vi "TEMP MOVE BIAS.vi"(0 "ScanQ in":refnum<queue>, 2 "Translation":cluster{"x":dbl, "y":dbl}, 5 "x":dbl, 7 "Boolean":bool, 9 "y":dbl, 11 "error in (no error)":errorcluster) -> (4 "ScanQ out":refnum<queue>, 6 "X (m)":sgl, 10 "Y (m)":sgl, 15 "error out":errorcluster)   [LabVIEW 2025]
uses:
  Labview-File/STM-Auto-Project Testing/STM-Auto-Project (Trial 2)/QMH CTLS/Scan_Params (QMH).ctl
  <userlib>/Nanonis Prog Interface V5e/Nanonis Prog Interface.lvlib
  Labview-File/STM-Auto-Project Testing/STM-Auto-Project (Trial 2)/QMH CTLS/Bias Cont QMH.ctl
panel:
  in  "Bias in":T1 {"Final Y (m)" format="%.3p"; "Final X (m)" format="%.3p"}
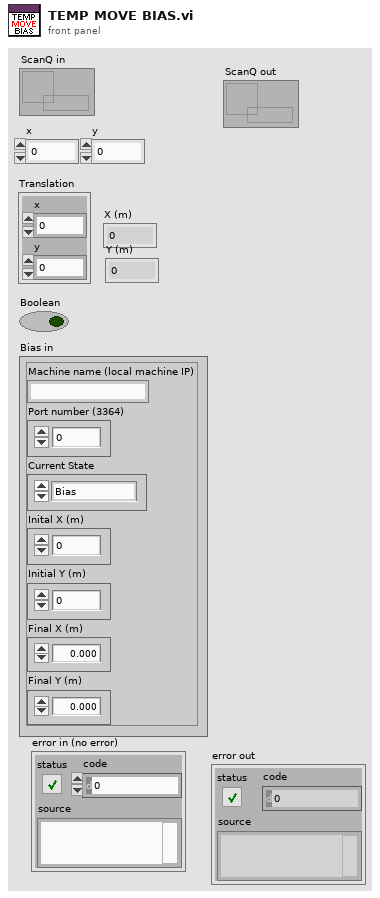
[diagram p1: front panel]
types:
  T1 = typedef "Bias Cont QMH.ctl" = cluster{"Machine name (local machine IP)":string, "Port number (3364)":u32, "Current State":enum16{"Bias", "Stop"}, "Inital X (m)":dbl, "Initial Y (m)":dbl, "Final X (m)":sgl, "Final Y (m)":sgl}
  T2 = enum16{"1. BIAS", "2. INIT_SCAN", "3. SCAN_IDLE", "4. INTER_SCAN", "5. NEW_COORDS_&_FRAME", "6. FINAL_SCAN", "7. POLL_BIAS", "8. Z-CONT.", "9. STOP"}
  T3 = typedef "Scan_Params (QMH).ctl" = cluster{"Setpoint (I)":dbl[], "Bias (V)":dbl[], "Number of scans":u8, "Port number (3364)":u32, "Avoid zero threshold (V)":dbl, "Current State":enum16{"1. BIAS", "2. INIT_SCAN", "3. SCAN_IDLE", "4. INTER_SCAN", "5. NEW_COORDS_&_FRAME", "6. FINAL_SCAN", "7. STOP"}}
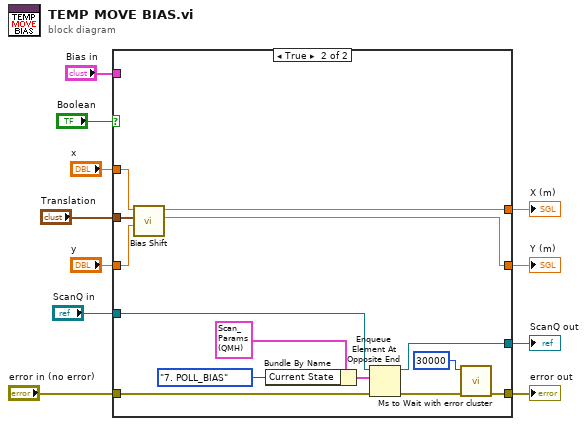
[diagram p0: block diagram]
diagram:
  n1 = case shown="True" "Boolean" {
    tunnel: "Translation" -> [_ w25]
    tunnel: "ScanQ in" -> [w15 w28]
    tunnel: [w15 w29] -> w8
    tunnel: [w14 w17] -> w9
    tunnel: "error in (no error)" -> [w14 w26]
    tunnel: [w13 w24] -> w4
    tunnel: "Bias in" -> [_ _]
    tunnel: [w12 w22] -> w3
    tunnel: "x" -> [w13 w21]
    tunnel: "y" -> [w12 w20]
    frame False {
    }
    frame True {
      n2 = call "Bias Shift.vi"("Initial Y"=w20, "Translation (m)"=w25, "Initial X"=w21) -> ("Final Y (m)"=w22:sgl, "FInal X (m)"=w24:sgl)  [unwired: 7 in]
      n3 = Bundle By Name(cluster=T3 {"Setpoint (I)"=[], "Bias (V)"=[], "Number of scans"=1, "Port number (3364)"=3364, "Avoid zero threshold (V)"=0.004999999888241291, "Current State"=enum."1. BIAS"} ("element"), "Current State"=T2."7. POLL_BIAS") -> (w23:T3)
      n4 = Enqueue Element At Opposite End(queue=w28, element=w23, error in (no error)=w26) -> (queue out=w29:refnum<queue>, error out=w18:errorcluster)  [unwired: 1 in, 1 out]
      n5 = call <userlib>:"Ms to Wait with error cluster.vi"("error in (no error)"=w18, "milliseconds to wait"=u32 30000) -> ("error out"=w17:errorcluster)  [unwired: 4 in, 1 out]
    }
  }
  "error out" <- w9
  "ScanQ out" <- w8
  "X (m)" <- w4
  "Y (m)" <- w3
